vi "Broken Rotor Bar Harmonics.vi"   [LabVIEW 2016, in "NI_EP_Motor Monitoring.lvlib"]
doc: "Calculates the sideband harmonics to detect broken rotor bars. You must manually select the polymorphic instance you want to use."
uses:
  <vilib>/addons/Electrical Power/Motor Monitoring/NI_EP_Motor Monitoring.lvlib
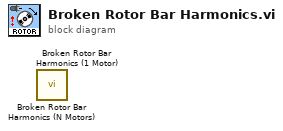
[diagram p0: block diagram]
diagram:
  n1 = call <vilib>:"Broken Rotor Bar Harmonics (N Motors).vi"() -> ()  [unwired: 12 in, 4 out]
  n2 = call <vilib>:"Broken Rotor Bar Harmonics (1 Motor).vi"() -> ()  [unwired: 12 in, 4 out]
